vi "Configure Measurement (Harmonics Distortion).vi"(0 "VISA resource name":refnum<visa-resource-name>, 1 "Enable Range Table (Disable)":bool, 2 "Enable Auto Fill Range Table (Disable)":bool, 5 "Harmonics Number (10)":i32=10, 7 "Enable Auto Sweep Time (T: Enable)":bool=TRUE, 9 "Manual Sweep Time (10 ms)":dbl=0.01 format="%#.6g", 11 "error in (no error)":errorcluster) -> (4 "VISA resource name out":refnum<visa-resource-name>, 15 "error out":errorcluster)   [LabVIEW 2014, in "Agilent ESA PSA Series.lvlib"]
doc: "Sets up the harmonic distortion measurement."
uses:
  Agilent ESA PSA Series.lvlib
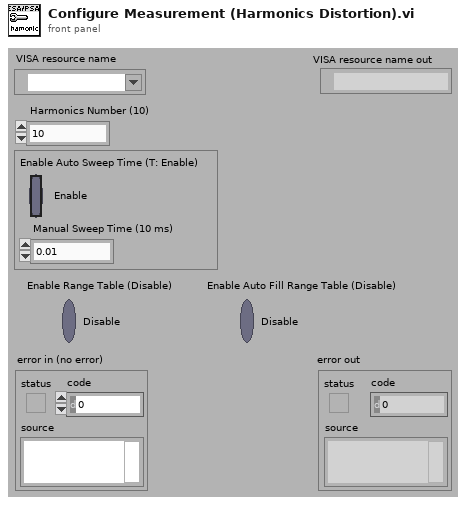
[diagram p1: front panel]
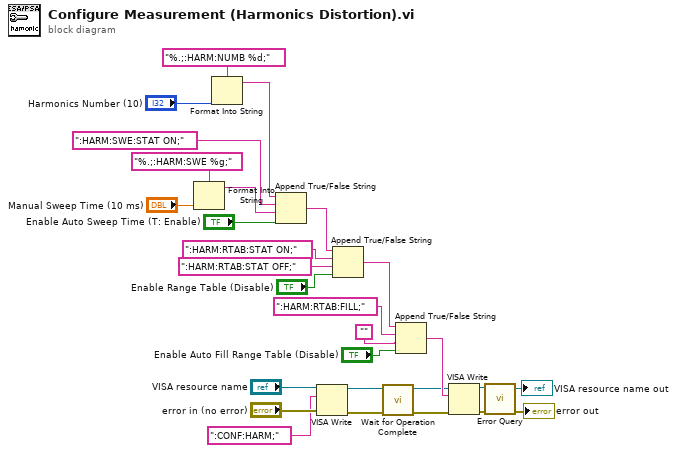
[diagram p0: block diagram]
diagram:
  n1 = Format Into String(format string="%.;:HARM:SWE %g;", "Manual Sweep Time (10 ms)") -> (resulting string=w22:string)  [unwired: 2 in, 1 out]
  n2 = Format Into String(format string="%.;:HARM:NUMB %d;", "Harmonics Number (10)") -> (resulting string=w10:string)  [unwired: 2 in, 1 out]
  n3 = Append True/False String(1:"Enable Auto Sweep Time (T: Enable)", 2:w22, 3:":HARM:SWE:STAT ON;" ("true string"), 4:w10) -> (0:w11:string)
  n4 = VISA Write(VISA resource name="VISA resource name", write buffer=":CONF:HARM;" ("initial string"), error in (no error)="error in (no error)") -> (VISA resource name out=w4:refnum<visa-resource-name>, error out=w3:errorcluster)  [unwired: 1 out]
  n5 = Append True/False String(1:"Enable Range Table (Disable)", 2:":HARM:RTAB:STAT OFF;" ("false string"), 3:":HARM:RTAB:STAT ON;" ("true string"), 4:w11) -> (0:w16:string)
  n6 = call "Wait for Operation Complete.vi"("error in (no error)"=w3, "VISA resource name"=w4) -> ("error out"=w2:errorcluster, "VISA resource name out"=w1:refnum<visa-resource-name>)  [unwired: 8 in]
  n7 = Append True/False String(1:"Enable Auto Fill Range Table (Disable)", 2:"", 3:":HARM:RTAB:FILL;" ("true string"), 4:w16) -> (0:w12:string)
  n8 = VISA Write(VISA resource name=w1, write buffer=w12, error in (no error)=w2) -> (VISA resource name out=w9:refnum<visa-resource-name>, error out=w8:errorcluster)  [unwired: 1 out]
  n9 = call "Error Query.vi"("error in (no error)"=w8, "VISA resource name"=w9) -> ("error out"=→"error out":errorcluster, "VISA resource name out"=→"VISA resource name out":refnum<visa-resource-name>)  [unwired: 6 in, 2 out]
